vi "Command.vi"(8 "error in (no error)":errorcluster, 10 "command":string, 11 "Comdel in":refnum<class "PL Comdel CX.lvclass">) -> (0 "error out":errorcluster, 2 "response data":string, 3 "Comdel out":refnum<class "PL Comdel CX.lvclass">)   [LabVIEW 2015, in "PL Comdel CX.lvclass"]
doc: "Sends <b>command</b> to device and returns <b>response data</b>."
uses:
  PL Comdel CX.lvclass
  PL Comdel CX.lvclass/PL Comdel CX.ctl
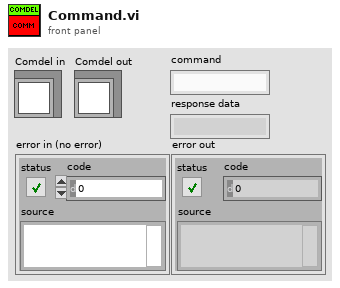
[diagram p1: front panel]
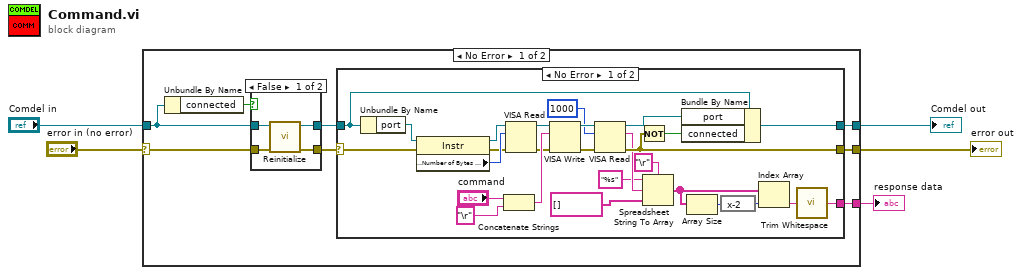
[diagram p0: block diagram]
diagram:
  n1 = case shown="No Error" "error in (no error)" {
    selector: "error in (no error)" -> [w11 w50]
    tunnel: "Comdel in" -> [w12 w49]
    tunnel: [w8 w50] -> w2
    tunnel: [w7 w49] -> w3
    tunnel: [w6 _] -> w1
    frame No Error {
      n2 = Unbundle By Name(w12) -> ("connected"=w13:bool)
      n3 = case shown="False" w13 {
        tunnel: w12 -> [w46 w48]
        tunnel: w11 -> [w45 w47]
        tunnel: [w44 w48] -> w9
        tunnel: [w43 w47] -> w10
        frame False {
          n4 = call "Reinitialize.vi"("error in (no error)"=w45, "Comdel in"=w46) -> ("error out"=w43:errorcluster, "Comdel out"=w44:refnum<class "PL Comdel CX.lvclass">)  [unwired: 8 in]
        }
        frame True {
        }
      }
      n5 = case shown="No Error" w10 {
        selector: w10 -> [w15 w42]
        tunnel: w9 -> [w34 w41]
        tunnel: [w30 w42] -> w8
        tunnel: [w31 w41] -> w7
        tunnel: [w29 _] -> w6
        frame No Error {
          n6 = Unbundle By Name(w34) -> ("port"=w16:refnum<visa-resource-name>)
          n7 = property class="Instr"(reference=w16, error in=w15) -> (reference out=w19:refnum<visa-resource-name>, error out=w14:errorcluster, "Serial Settings:Number of Bytes at Serial Port"=w20:u32)
          n8 = Concatenate Strings("command", "\r" ("string")) -> (w36:string)
          n9 = VISA Read(VISA resource name=w19, byte count=w20, error in (no error)=w14) -> (VISA resource name out=w18:refnum<visa-resource-name>, error out=w17:errorcluster)  [unwired: 2 out]
          n10 = VISA Write(VISA resource name=w18, write buffer=w36, error in (no error)=w17) -> (VISA resource name out=w40:refnum<visa-resource-name>, error out=w39:errorcluster)  [unwired: 1 out]
          n11 = VISA Read(VISA resource name=w40, byte count=u32 1000, error in (no error)=w39) -> (VISA resource name out=w33:refnum<visa-resource-name>, read buffer=w28:string, error out=w30:errorcluster)  [unwired: 1 out]
          n12 = Not(x=w30) -> (.not. x?=w32:bool)
          n13 = Spreadsheet String To Array(delimiter (Tab)="\r", format string="%s", spreadsheet string=w28, array type (2D Dbl)=string[] []) -> (array=w24:string[])
          n14 = Bundle By Name(cluster=w34, "port"=w33, "connected"=w32) -> (w31:refnum<class "PL Comdel CX.lvclass">)
          n15 = Array Size(array=w24) -> (size(s)=w22:i32)
          n16 = expression code="x-2"(w22) -> (w21:i32)
          n17 = Index Array(array=w24, index=w21) -> (element=w23:string)
          n18 = call <vilib>:"Trim Whitespace.vi"("string"=w23) -> ("trimmed string"=w29:string)  [unwired: 1 in]
        }
        frame Error {
        }
      }
    }
    frame Error {
    }
  }
  "Comdel out" <- w3
  "response data" <- w1
  "error out" <- w2
